vi "tcp.vi"() -> ()   [LabVIEW 2018]
panel:
  in  "stop":bool
  out "No error":errorcluster
  out "Message from Server":string
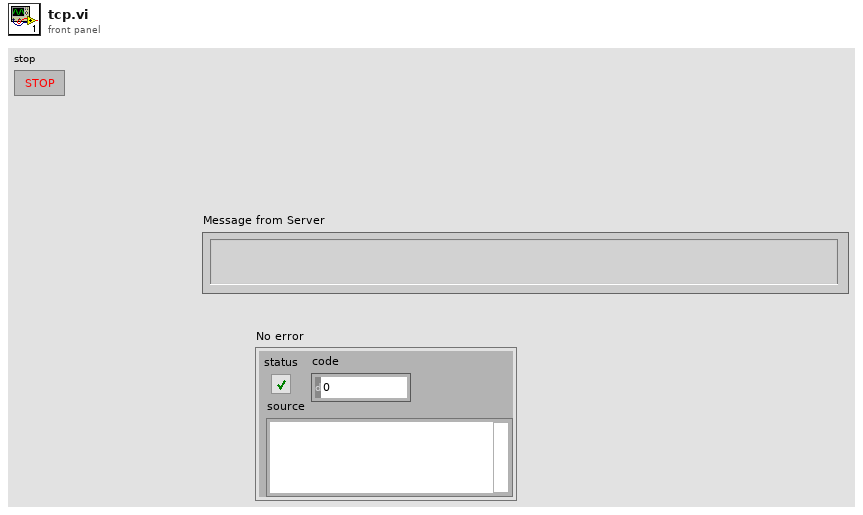
[diagram p1: front panel]
types:
  T1 = enum16{"Standard", "Buffered", "CRLF", "Immediate"}
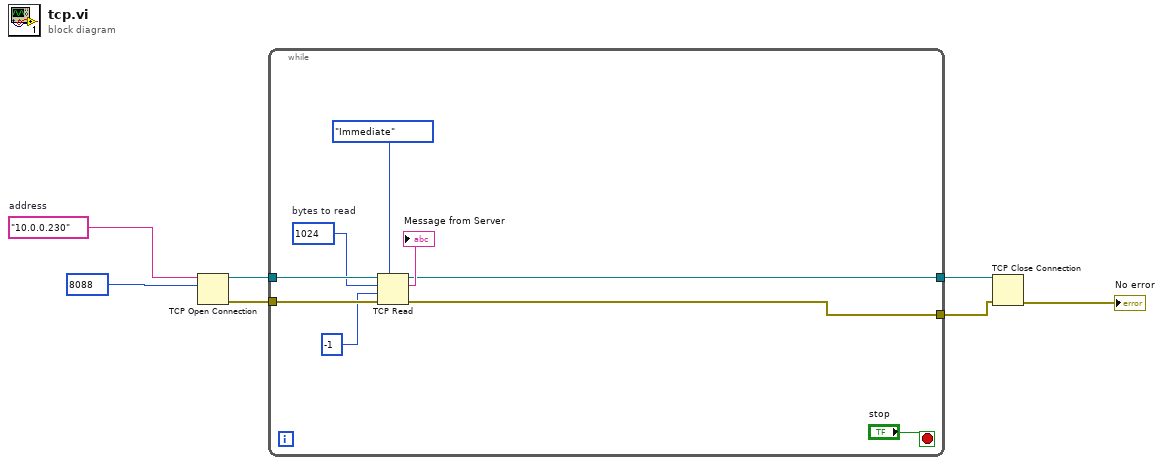
[diagram p0: block diagram]
diagram:
  w7 = "10.0.0.230"  # address
  n1 = TCP Open Connection(address=w7, remote port or service name=u16 8088) -> (connection ID=w4:refnum<k5>, error out=w5:errorcluster)  [unwired: 3 in]
  n2 = while {
    tunnel: w5 -> [w16]
    tunnel: w4 -> [w15]
    tunnel: [w9] -> w3
    tunnel: [w8] -> w2
    stop <- "stop" stop-if-true
    w13 = 1024  # bytes to read
    n3 = TCP Read(connection ID=w15, bytes to read=w13, error in (no error)=w16, 7:T1."Immediate" ("mode (standard)"), 9:-1 ("timeout ms (25000)")) -> (connection ID out=w8:refnum<k5>, data out=→"Message from Server":string, error out=w9:errorcluster)
  }
  n4 = TCP Close Connection(connection ID=w2, error in (no error)=w3) -> (error out=→"No error":errorcluster)  [unwired: 1 in, 1 out]
